vi "Analog Read Pin.vi"(0 "Arduino Resource":T1={"VISA resource"="COM11", "Board Type"=enum."Arduino Uno", "Connection Type"=enum."USB / Serial", "Bytes Per Packet (15)"=15}, 7 "Analog Pin":u8, 11 "error in":errorcluster) -> (4 "Arduino Resource":T1={"VISA resource"="COM11", "Board Type"=enum."Arduino Uno", "Connection Type"=enum."USB / Serial", "Bytes Per Packet (15)"=15}, 8 "Voltage":dbl(knob) scale=0.0..5.0, 15 "error out":errorcluster)   [LabVIEW 2011, in "LabVIEW Interface for Arduino.lvlib"]
doc: "Reads the analog voltage on the selected Arduino analog input pin (A0 - A5)."
uses:
  <vilib>/LabVIEW Interface for Arduino/LabVIEW Interface for Arduino.lvlib
  <vilib>/LabVIEW Interface for Arduino/Private/Type Defs/Arduino Resource.ctl
  <vilib>/LabVIEW Interface for Arduino/Private/Type Defs/Board Type.ctl
  <vilib>/LabVIEW Interface for Arduino/Private/Type Defs/Command.ctl
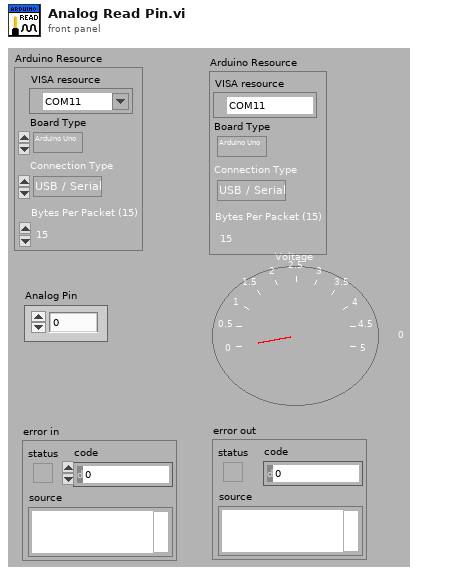
[diagram p1: front panel]
types:
  T1 = typedef "LabVIEW Interface for Arduino.lvlib/Arduino Resource.ctl" = cluster{"VISA resource":refnum<visa-resource-name>, "Board Type":T2, "Connection Type":enum8{"USB / Serial"}, "Bytes Per Packet (15)":u8}
  T2 = typedef "LabVIEW Interface for Arduino.lvlib/Board Type.ctl" = enum16{"Arduino Uno", "Dimuelanove w/Atmega 328", "Mega 2560", "Chipkit Uno32", "Chipkit Max32"}
  T3 = typedef "LabVIEW Interface for Arduino.lvlib/Command.ctl" = enum8{"setArduinoMode", "flushSerial", "setPinMode", "digitalWritePin", "digitalWritePort", "tone", "digitalReadPin", "digitalReadPort", "analogReadPin", "analogReadPort", "pwmWritePin", "pwmWritePort", "sevenSegment_Configure", "sevenSegment_Write", "I2C Init", "I2C Write", "I2C Read", "SPI Init", "SPI Set Bit Order", "SPI Set Clock Divider", "SPI Set Data Mode", "SPI Send / Receive", "SPI Close", "Servo Set Num Servos", "Servo Config Servo", "Servo Write Angle", "Servo Read Angle", "Servo Write Pulse Width", "Servo Read Pulse Width", "Servo Detach", "LCD Init", "LCD Set Size", "LCD Set Cursor Mode", "LCD Clear", "LCD Set Cursor Position", "LCD Print", "LCD Display Power", "LCD Scroll Display", "LCD Autoscroll", "LCD Print Direction", "LCD Create Custom Char", "LCD Print Custom Char", "contAcqOn", "contAcqOff", "getFirmwareVersion", "FiniteSampleStart"}
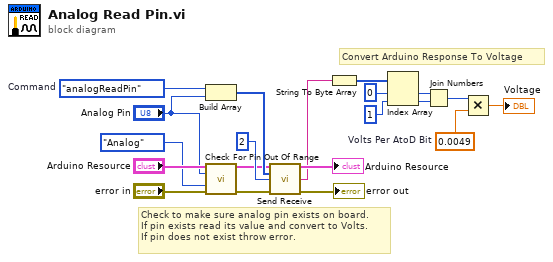
[diagram p0: block diagram]
diagram:
  w17 = 0.0049  # Volts Per AtoD Bit
  w15 = Command."analogReadPin"  # Command
  # "Check to make sure analog pin exists on board.\nIf pin exists read its value and convert to Volts.\nIf pin does not exist throw error."
  # "Convert Arduino Response To Voltage"
  n1 = Build Array(w15, "Analog Pin") -> (w14:u8[])
  n2 = call <vilib>:"Check For Pin Out Of Range.vi"("Arduino Resource"="Arduino Resource", "User Pin Number"="Analog Pin", "Pin Type"=enum16{"Analog", "Digital"}."Analog", "error in"="error in") -> ("Arduino Resource"=w6:T1, "error out"=w8:errorcluster)  [unwired: 10 in]
  n3 = call <vilib>:"Send Receive.vi"("Arduino Resource"=w6, "Data"=w14, "Bytes To Read (0)"=u32 2, "error in"=w8) -> ("Arduino Resource"=→"Arduino Resource":T1, "Read Buffer"=w10:string, "error out"=→"error out":errorcluster)  [unwired: 9 in]
  n4 = String To Byte Array(string=w10) -> (unsigned byte array=w20:u8[])
  n5 = Index Array(array=w20, index #1=0 ("index"), index #2=1 ("index")) -> (element #1=w4:u8, element #2=w3:u8)
  n6 = Join Numbers(hi=w4, lo=w3) -> ((hi.lo)=w2:u16)
  n7 = Multiply(x=w2, y=w17) -> (x*y=→"Voltage":dbl)
